vi "text2word.vi"(11 "Text":string) -> (3 "Number":i32)   [LabVIEW 2021, in "2023.lvlib"]
uses:
  2023/2023.lvlib
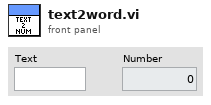
[diagram p1: front panel]
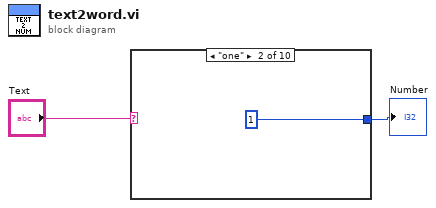
[diagram p0: block diagram]
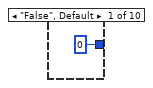
[diagram p2: hidden frame]
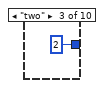
[diagram p3: hidden frame]
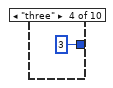
[diagram p4: hidden frame]
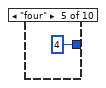
[diagram p5: hidden frame]
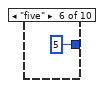
[diagram p6: hidden frame]
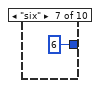
[diagram p7: hidden frame]
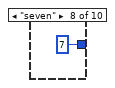
[diagram p8: hidden frame]
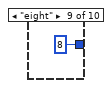
[diagram p9: hidden frame]
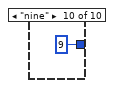
[diagram p10: hidden frame]
diagram:
  n1 = case shown="\"one\"" "Text" {
    tunnel: [0 ("default (0 I32)") 1 ("default (0 I32)") 2 ("default (0 I32)") 3 ("default (0 I32)") 4 ("default (0 I32)") 5 ("default (0 I32)") 6 ("default (0 I32)") 7 ("default (0 I32)") 8 ("default (0 I32)") 9 ("default (0 I32)")] -> w2
    frame "False", Default {
    }
    frame "one" {
    }
    frame "two" {
    }
    frame "three" {
    }
    frame "four" {
    }
    frame "five" {
    }
    frame "six" {
    }
    frame "seven" {
    }
    frame "eight" {
    }
    frame "nine" {
    }
  }
  "Number" <- w2
